vi "SUB-프런트패널 종료.vi"   [LabVIEW 2015]
types:
  T1 = enum32{"invalid app kind", "Development System", "Run Time System", "Student Edition", "Embedded LabVIEW", "Evaluation", "Custom"}
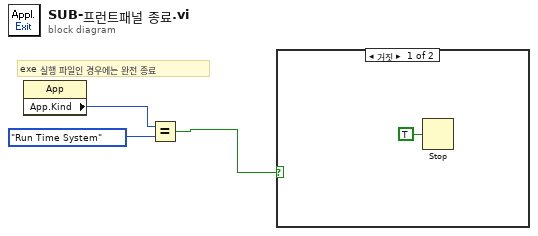
[diagram p0: block diagram]
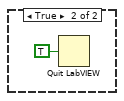
[diagram p2: hidden frame]
diagram:
  # "exe 실행 파일인 경우에는 완전 종료"
  n1 = property class="App"() -> ("App.Kind"=w2:T1)  [unwired: 2 in, 2 out]
  n2 = Equal?(x=w2, y=T1."Run Time System" ("Application:Kind")) -> (x = y?=w1:bool)
  n3 = case shown="거짓" w1 {
    frame False {
      n4 = Stop(stop? (T)=TRUE ("정지? (참)")) -> ()
    }
    frame True {
      n5 = Quit LabVIEW(quit? (T)=TRUE ("종료? (참)")) -> ()
    }
  }
